vi "XML Script - Frame.vi"(0 "x":i32=-1, 1 "y":i32=-1, 2 "out":i32=-1, 3 "default":bool, 4 "diagram (XML)":string, 6 "name":string, 8 "value":string, 9 "prefix (name)":string, 10 "in":i32=-1, 11 "index":i32) -> (5 "name (wire source)":string, 7 "XML Script Command - Frame":string)   [LabVIEW 2020]
uses:
  <vilib>/_script/XML Scripting/XML Script Tag.ctl
  <vilib>/_script/XML Scripting/XML Script Attribute.ctl
panel:
  # "position"
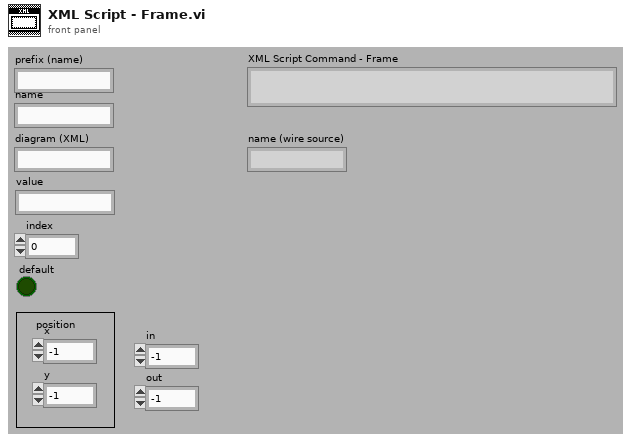
[diagram p1: front panel]
types:
  T1 = typedef "XML Script Attribute.ctl" = enum16{"name", "style", "path", "position", "in", "out", "width", "height", "index", "value", "default", "location", "offset", "typeindex", "size", "source", "destination", "indicator", "type", "controlname", "label", "conpaneidx", "mode", "description", "hasCondTerm", "linkIdentity", "caseselectortype", "concatInputs", "inName", "instantiationpath", "loopCondition", "IndexMode", "formulaInputs", "formulaOutputs", "msnFuncName", "msnIsDynamic", "msnIsODEUserFunction", "ignoreSearchDialog"}
  T2 = typedef "XML Script Tag.ctl" = enum16{"Script", "Function", "SubVI", "GrowableFunction", "Structure", "MultiframeStructure", "Frame", "Tunnel", "ShiftRegister", "Constant", "Control", "Terminal", "Wire", "StaticVIReference", "ControlTerminal", "CompoundArithmetic", "FlatSequence", "FlatSequenceFrame", "MathScriptCallByRef", "BuildArray", "GenericSubVI", "MathScriptNode"}
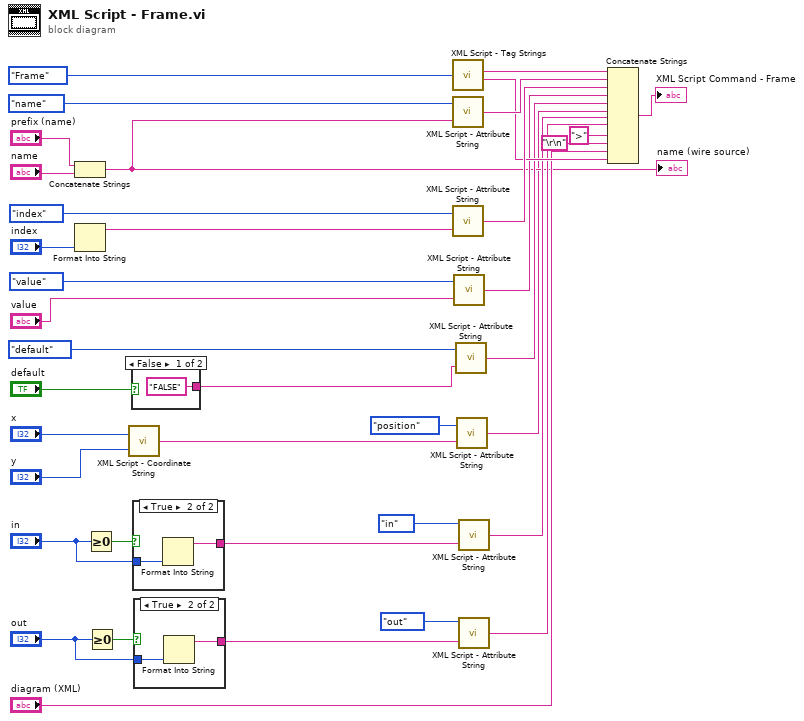
[diagram p0: block diagram]
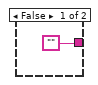
[diagram p2: hidden frame]
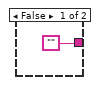
[diagram p3: hidden frame]
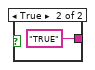
[diagram p4: hidden frame]
diagram:
  n1 = Concatenate Strings("prefix (name)", "name") -> (w6:string)
  "name (wire source)" <- w6
  n2 = Format Into String("index") -> (resulting string=w28:string)  [unwired: 3 in, 1 out]
  n3 = Greater Or Equal To 0?(x="in") -> (x >= 0?=w15:bool)
  n4 = Greater Or Equal To 0?(x="out") -> (x >= 0?=w18:bool)
  n5 = call <vilib>:"XML Script - Coordinate String.vi"("y"="y", "x"="x") -> ("(x,y)"=w4:string)
  n6 = case shown="False" "default" {
    tunnel: ["FALSE" "TRUE"] -> w21
    frame False {
    }
    frame True {
    }
  }
  n7 = case shown="True" w15 {
    tunnel: "in" -> [_ w43]
    tunnel: ["" w42] -> w17
    frame False {
    }
    frame True {
      n8 = Format Into String(w43) -> (resulting string=w42:string)  [unwired: 3 in, 1 out]
    }
  }
  n9 = case shown="True" w18 {
    tunnel: "out" -> [_ w46]
    tunnel: ["" w45] -> w20
    frame False {
    }
    frame True {
      n10 = Format Into String(w46) -> (resulting string=w45:string)  [unwired: 3 in, 1 out]
    }
  }
  n11 = call <vilib>:"XML Script - Tag Strings.vi"("XML Script Tag"=XML_Script_Tag."Frame") -> ("XML String - Begin Tag"=w37:string, "XML String - End Tag"=w31:string)  [unwired: 2 in]
  n12 = call <vilib>:"XML Script - Attribute String.vi"("Attribute String"=w6, "XML Script Attribute"=XML_Script_Attribute."name") -> ("XML Script - Attribute String"=w34:string)
  n13 = call <vilib>:"XML Script - Attribute String.vi"("Attribute String"=w28, "XML Script Attribute"=XML_Script_Attribute."index") -> ("XML Script - Attribute String"=w32:string)
  n14 = call <vilib>:"XML Script - Attribute String.vi"("Attribute String"="value", "XML Script Attribute"=XML_Script_Attribute."value") -> ("XML Script - Attribute String"=w10:string)
  n15 = call <vilib>:"XML Script - Attribute String.vi"("Attribute String"=w21, "XML Script Attribute"=XML_Script_Attribute."default") -> ("XML Script - Attribute String"=w11:string)
  n16 = call <vilib>:"XML Script - Attribute String.vi"("Attribute String"=w4, "XML Script Attribute"=XML_Script_Attribute."position") -> ("XML Script - Attribute String"=w1:string)
  n17 = call <vilib>:"XML Script - Attribute String.vi"("Attribute String"=w17, "XML Script Attribute"=XML_Script_Attribute."in") -> ("XML Script - Attribute String"=w12:string)
  n18 = call <vilib>:"XML Script - Attribute String.vi"("Attribute String"=w20, "XML Script Attribute"=XML_Script_Attribute."out") -> ("XML Script - Attribute String"=w13:string)
  n19 = Concatenate Strings(w37, w34, w32, w10, w11, w1, w12, w13, ">" ("string"), "\r\n", "diagram (XML)", w31) -> (→"XML Script Command - Frame":string)
